vi "Write.vi"(8 "error in (no error)":errorcluster, 10 "Cluster":variant, 11 "Cluster in":refnum<class "Cluster.lvclass">) -> (0 "error out":errorcluster, 1 "Success?":bool, 3 "Cluster out":refnum<class "Cluster.lvclass">)   [LabVIEW 2020, in "Data.lvlib" / "Cluster.lvclass"]
doc: "Write Cluster using 'Wrap in Generic'"
uses:
  Cluster.lvclass
  Cluster.lvclass/Cluster.ctl
  <vilib>/Utility/Data Type/NI_Data Type.lvlib
  Data.lvlib
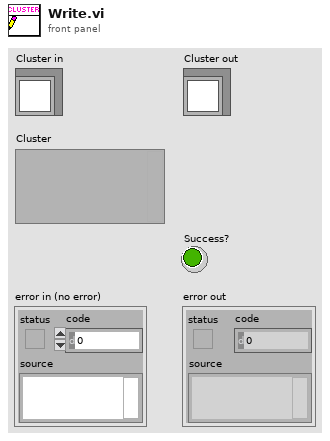
[diagram p1: front panel]
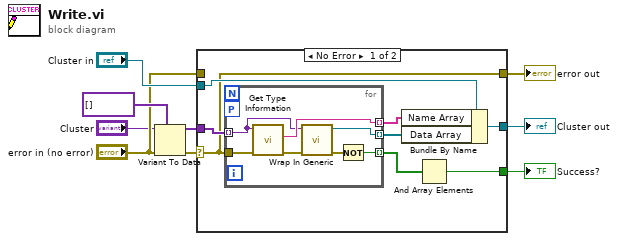
[diagram p0: block diagram]
diagram:
  n1 = Variant To Data(error in="error in (no error)", type=variant[] [] ("Cluster"), Variant="Cluster") -> (data=w1:variant[], error out=w4:errorcluster)
  n2 = case shown="No Error" w4 {
    selector: w4 -> [w10 _]
    tunnel: [w10 w25] -> w9
    tunnel: [w12 w26] -> w7
    tunnel: "Cluster in" -> [w15 w26]
    tunnel: [w16 _] -> w6
    tunnel: "error in (no error)" -> [_ w25]
    tunnel: w1 -> [w11 _]
    frame No Error {
      n3 = for {
        tunnel: w10 -> [w24]
        tunnel: [w23] -> w14 mode=indexing
        tunnel: [w21] -> w13 mode=indexing
        tunnel: [w19] -> w17 mode=indexing
        workers-P: _ -> [_]
        tunnel: w11 -> [w20] mode=indexing
        n4 = call <vilib>:"Get Type Information.vi"("error in (no error)"=w24, "variant"=w20) -> ("error out"=w22:errorcluster, "name"=w23:string)  [unwired: 5 in, 3 out]
        n5 = call "Wrap In Generic.vi"("error in (no error)"=w22, "Data to Wrap"=w20) -> ("error out"=w18:errorcluster, "Generic Data"=w21:refnum<class "Generic Data.lvclass">)  [unwired: 8 in]
        n6 = Not(x=w18) -> (.not. x?=w19:bool)
      }
      n7 = Bundle By Name(cluster=w15, "Name Array"=w14, "Data Array"=w13) -> (w12:refnum<class "Cluster.lvclass">)
      n8 = And Array Elements(Boolean array=w17) -> (logical AND=w16:bool)
    }
    frame Error {
    }
  }
  "error out" <- w9
  "Cluster out" <- w7
  "Success?" <- w6
